vi "Flatten.vi"(8 "error in (no error)":errorcluster, 10 "Pretty Print?":bool, 11 "JSON Array in":refnum<class "JSON Array.lvclass">) -> (0 "error out":errorcluster, 2 "String":string)   [LabVIEW 2011, in "JSON Array.lvclass"]
doc: "Converts an <b>JSON array</b> into <b>String</b>. Use <b>Pretty Print?</b> to auto-indent and distribute the string over different lines.\n\nCopyright 2012 James David Powell, Shaun Rumbell and Ton Plomp\nMore information on http://lavag.org/topic/16217-cr-json-labview"
uses:
  JSON Array.lvclass
  JSON Array.lvclass/JSON Array.ctl
  JSON Value/JSON Value.lvclass
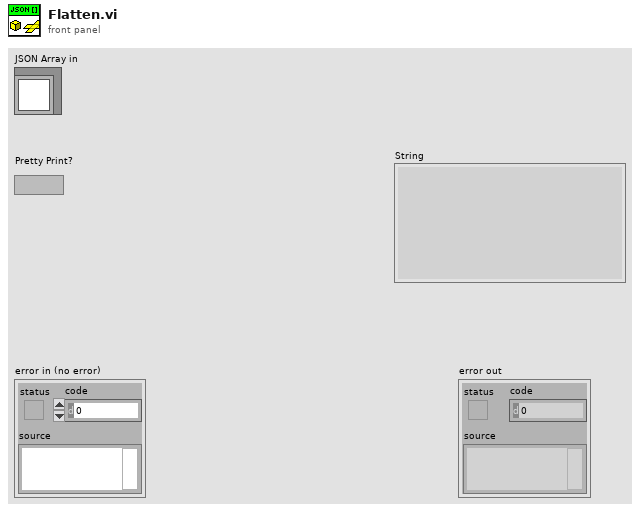
[diagram p1: front panel]
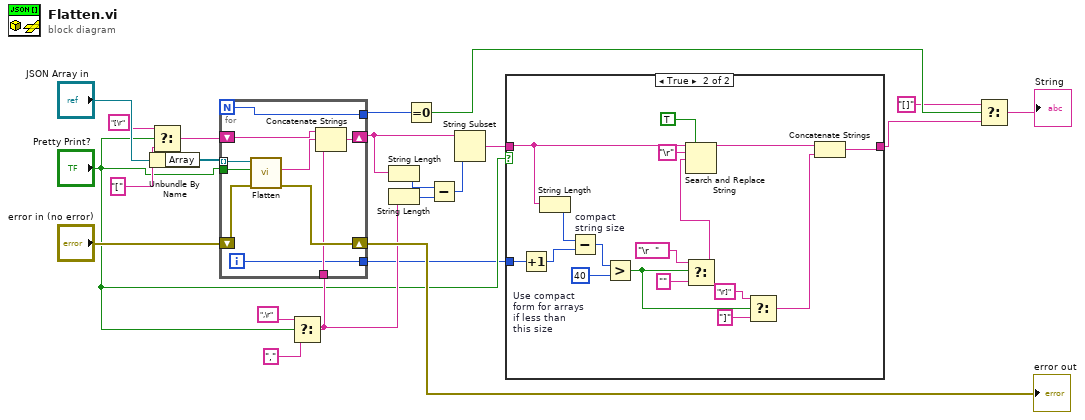
[diagram p0: block diagram]
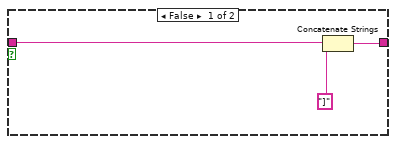
[diagram p2: hidden frame]
diagram:
  n1 = Unbundle By Name("JSON Array in") -> ("Array"=w21:refnum<class "JSON Value.lvclass">[])
  n2 = Select(t="[\r", s="Pretty Print?", f="[") -> (s? t:f=w10:string)
  n3 = Select(t=",\r" ("string"), s="Pretty Print?", f="," ("string")) -> (s? t:f=w4:string)
  n4 = for {
    N -> [w26]
    tunnel: w21 -> [w32] mode=indexing
    shift-right: [w31] -> w14
    shift-left: w10 -> [w30]
    shift-right: [w28] -> w19
    shift-left: "error in (no error)" -> [w29]
    tunnel: "Pretty Print?" -> [w27]
    tunnel: [w26] -> w17
    tunnel: w4 -> [w24]
    tunnel: [w23] -> w1
    i -> [w23]
    n5 = call-dynamic "Flatten.vi"("error in (no error)"=w29, "Pretty Print?"=w27, "JSON Value in"=w32) -> ("error out"=w28:errorcluster, "String"=w25:string)  [unwired: 7 in]
    n6 = Concatenate Strings(w30, w25, w24) -> (w31:string)
  }
  "error out" <- w19
  n7 = String Length(string=w14) -> (length=w13:i32)
  n8 = String Length(string=w4) -> (length=w12:i32)
  n9 = Equal To 0?(x=w17) -> (x = 0?=w18:bool)
  n10 = Subtract(x=w13, y=w12) -> (x-y=w11:i32)
  n11 = String Subset(string=w14, length (rest)=w11) -> (substring=w8:string)  [unwired: 1 in]
  n12 = case shown="True" "Pretty Print?" {
    tunnel: w8 -> [w33 w48]
    tunnel: [w34 w49] -> w2
    tunnel: w1 -> [_ w47]
    frame False {
      n13 = Concatenate Strings(w33, "]" ("substring (\"\")")) -> (w34:string)
    }
    frame True {
      w43 = 40  # Use compact form for arrays  if less than  this size
      n14 = Increment(x=w47) -> (x+1=w45:i32)
      n15 = String Length(string=w48) -> (length=w46:i32)
      n16 = Subtract "compact \nstring size"(x=w46, y=w45) -> (x-y=w44:i32)
      n17 = Greater?(x=w44, y=w43) -> (0:w39:bool)
      n18 = Select(t="\r  " ("search string"), s=w39, f="") -> (s? t:f=w40:string)
      n19 = Search and Replace String(replace all?=TRUE ("replace all? (F)"), input string=w48, search string="\r", replace string=w40) -> (result string=w50:string)  [unwired: 4 in, 3 out]
      n20 = Select(t="\r]" ("search string"), s=w39, f="]") -> (s? t:f=w36:string)
      n21 = Concatenate Strings(w50, w36) -> (w49:string)
    }
  }
  n22 = Select(t="[]", s=w18, f=w2) -> (s? t:f=→"String":string)
